vi "CLUST_AUTO_SwitchBools.vi"() -> ()   [LabVIEW 2017]
uses:
  CLUSTER_AUTO_switchBools.ctl
panel:
  in  "Cluster":T1
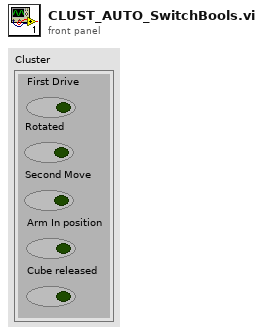
[diagram p1: front panel]
types:
  T1 = typedef "CLUSTER_AUTO_switchBools.ctl" = cluster{"First Drive":bool, "Rotated ":bool, "Second Move":bool, "Arm In position":bool, "Cube released":bool}
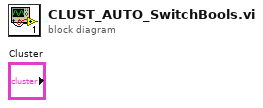
[diagram p0: block diagram]
diagram:
